vi "MT Generate Symbol Map (Rectangular).vi"(0 "symbol values":i32[][](array[numeric]), 5 "symbol amplitudes (I)":dbl[](array[numeric]), 7 "symbol amplitudes (Q)":dbl[](array[numeric]), 11 "error in (no error)":errorcluster, 13 "gain":dbl=1.0) -> (4 "symbol map":cdb[](array[numeric]) format="%.3f", 15 "error out":errorcluster)   [LabVIEW 2020, in "niDMT.lvlib"]
doc: "This polymorphic instance generates a symbol map with an input matrix of symbol values and I/Q symbol amplitude arrays that you specify. Use the <B>symbol map</B> parameter of the <B>system parameters</B> cluster to configure the operation of the demodulation and modulation VIs.\n\nThe <B>symbol values</B> matrix defines how the M-ary binary data are mapped to the discrete I/Q symbols on the constellation diagram. The optional <B>gain</B> parameter can be used to multiply the generated symbol map by a scalar value. The VI internally reads the <B>symbol values</B> matrix row-wise and uses the I/Q symbol amplitudes array values to assign the symbol amplitudes to each element in the row.\n\n<B>NOTE:</B> The number of rows in the symbol amplitudes matrix must exactly equal the length of the"
uses:
  <vilib>/addons/Modulation/niDMT.lvlib
  <vilib>/addons/Modulation/niAMT.lvlib
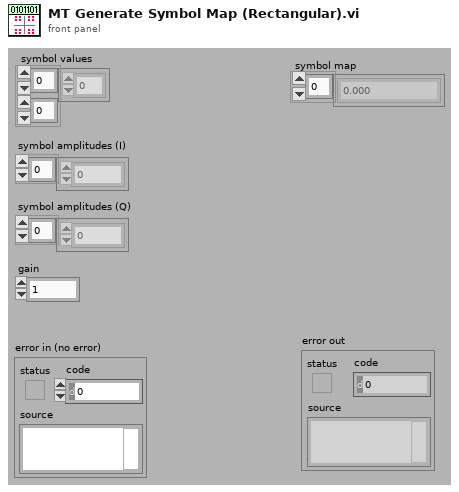
[diagram p1: front panel]
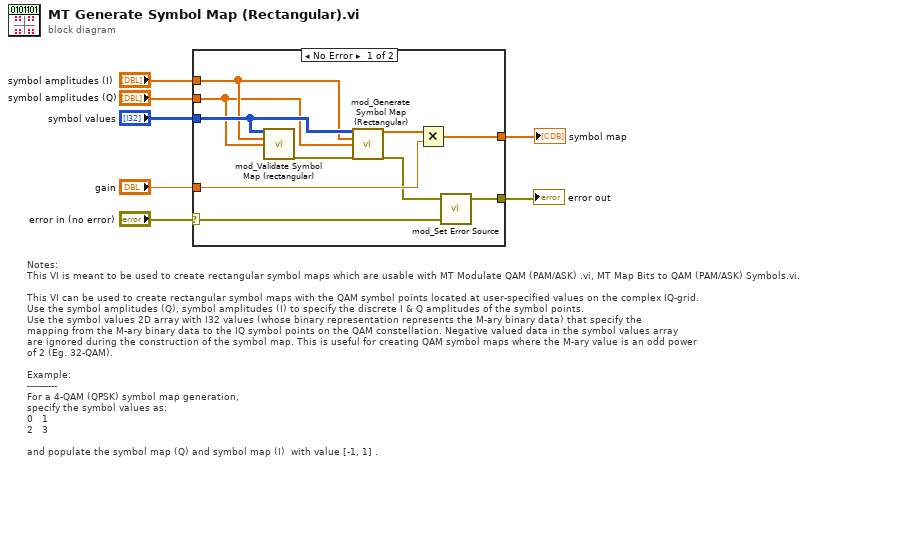
[diagram p0: block diagram]
diagram:
  # "Notes:\nThis VI is meant to be used to create rectangular symbol maps which are usable with MT Modulate QAM (PAM/ASK) .vi, MT Map Bits to QAM (PAM/ASK) Symbols.vi.\n\nThis VI can be used to create rectangular symbol maps with the QAM symbol points located at user-specified values on the complex IQ-grid.\nUse the symbol amplitudes (Q), symbol amplitudes (I) to specify the discrete I & Q amplitudes of the symbol points. \nUse the symbol values 2D array with I32 values (whose binary representation represents the M-ary binary data) that specify the \nmapping from the M-ary binary data to the IQ symbol points on the QAM constellation. Negative valued data in the symbol values array\nare ignored during the construction of the symbol map. This is useful for creating QAM symbol maps where the M-ary value is an odd power\nof 2 (Eg. 32-QAM).\n\nExample:\n----------\nFor a 4-QAM (QPSK) symbol map generation,\nspecify the symbol values as:\n0   1\n2   3\n\nand populate the symbol map (Q) and symbol map (I)  with value [-1, 1] ."
  n1 = case shown="No Error" "error in (no error)" {
    selector: "error in (no error)" -> [w14 _]
    tunnel: "symbol values" -> [w13 _]
    tunnel: "symbol amplitudes (I)" -> [w9 _]
    tunnel: [w15 _] -> w5
    tunnel: "gain" -> [w17 _]
    tunnel: [w10 _] -> w2
    tunnel: "symbol amplitudes (Q)" -> [w8 _]
    frame No Error {
      n2 = call <vilib>:"mod_Validate Symbol Map (rectangular).vi"("symbol values"=w13, "symbol amplitudes (I)"=w9, "symbol amplitudes (Q)"=w8) -> ("error out"=w12:errorcluster)  [unwired: 12 out]
      n3 = call <vilib>:"mod_Generate Symbol Map (Rectangular).vi"("symbol values"=w13, "symbol amplitudes (I)"=w9, "symbol amplitudes (Q)"=w8, "error in (no error)"=w12) -> ("symbol map"=w16:cdb[], "error out"=w11:errorcluster)  [unwired: 10 out]
      n4 = Multiply(x=w16, y=w17) -> (x*y=w15:cdb[])
      n5 = call <vilib>:"mod_Set Error Source.vi"("initial error in (no error)"=w14, "final error in (no error)"=w11) -> ("error out"=w10:errorcluster)  [unwired: 3 out]
    }
    frame Error {
    }
  }
  "symbol map" <- w5
  "error out" <- w2
